vi "preguntaAjustesPrevios.vi"(8 "error in (no error)":errorcluster, 11 "Equipo in":refnum<class "Equipo.lvclass">) -> (0 "error out":errorcluster, 2 "Si":bool, 3 "Equipo out":refnum<class "Equipo.lvclass">)   [LabVIEW 2019, in "Equipo.lvclass"]
uses:
  Equipo.lvclass
panel:
  in  "No":bool
  in  "Si":bool
  # "¿Desea realizar los Ajustes Previos?"
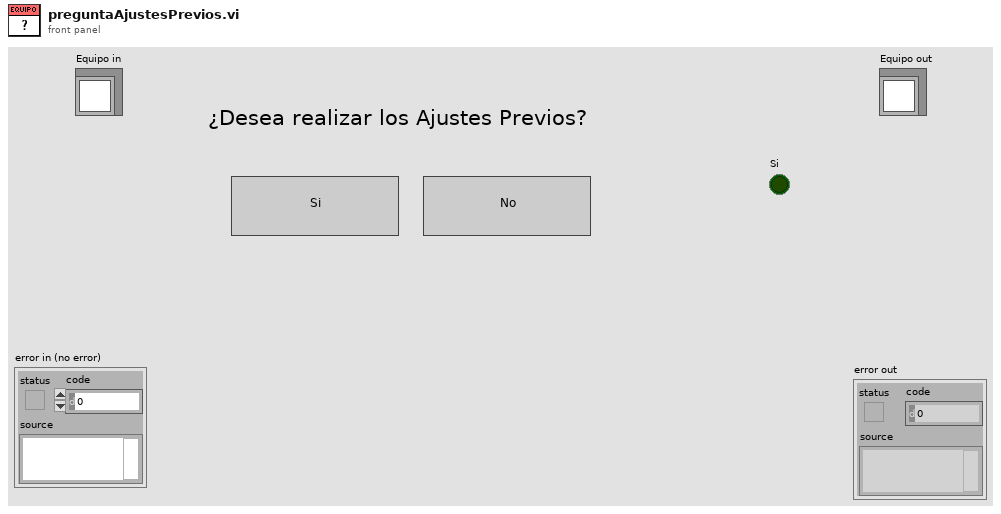
[diagram p1: front panel]
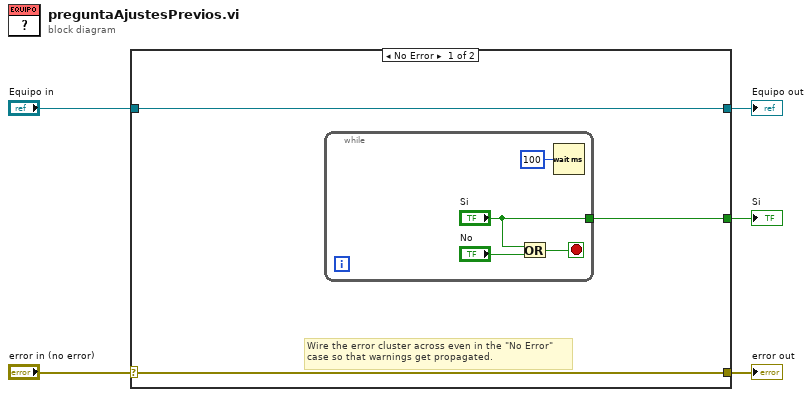
[diagram p0: block diagram]
diagram:
  n1 = case shown="No Error" "error in (no error)" {
    selector: "error in (no error)" -> [w7 w14]
    tunnel: [w7 w14] -> w4
    tunnel: [w8 w13] -> w2
    tunnel: "Equipo in" -> [w8 w13]
    tunnel: [w6 _] -> w1
    frame No Error {
      # "Wire the error cluster across even in the \"No Error\"\ncase so that warnings get propagated."
      n2 = while {
        tunnel: ["Si"] -> w6
        stop <- w11 stop-if-true
        n3 = Or(x="Si", y="No") -> (x .or. y?=w11:bool)
        n4 = Wait (ms)(milliseconds to wait=u32 100) -> ()  [unwired: 1 out]
      }
    }
    frame Error {
    }
  }
  "error out" <- w4
  "Equipo out" <- w2
  "Si" <- w1
